vi "ifr2025 Reverse Power Protection  .vi"(8 "error in (no error)":errorcluster {"code" format="%.0x"}, 11 "instrument handle":refnum<visa-resource-name>) -> (0 "error out":errorcluster {"code" format="%.0x"}, 1 "RPP Count":i16, 2 "RPP Tripped":i16, 3 "instrument handle out":refnum<visa-resource-name>)   [LabVIEW 2009]
doc: "Returns information about the reverse power protection circuit."
uses:
  Ifr2025_32.dll
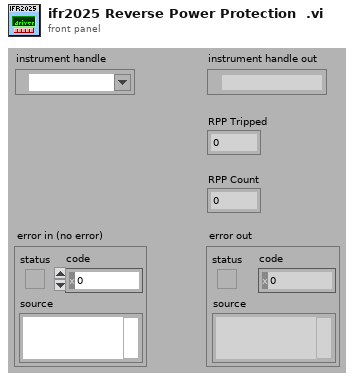
[diagram p1: front panel]
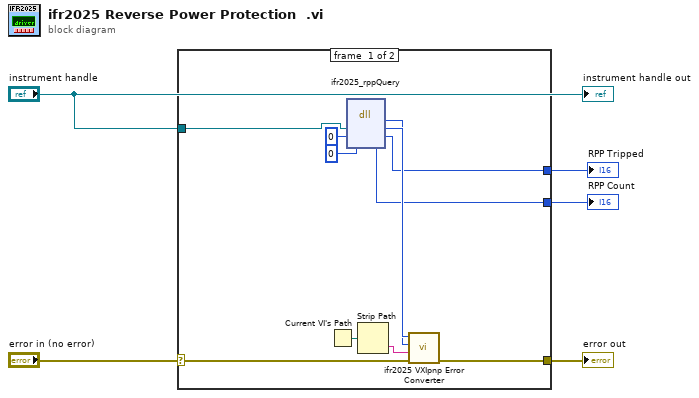
[diagram p0: block diagram]
diagram:
  n1 = case shown="No Error" "error in (no error)" {
    selector: "error in (no error)" -> [w11 w17]
    tunnel: [w10 w17] -> w5
    tunnel: "instrument handle" -> [w15 _]
    tunnel: [w8 _] -> w2
    tunnel: [w6 _] -> w1
    frame #0 {
      n2 = Current VI's Path() -> (path=w16:path)
      n3 = dll-call lib="P:/inst/Marconi 2024 Signal Generator/source/labview/ifr2025/ifr2025/ifr2025_*.*" fn="ifr2025_rppQuery"("vi"=w15, "RPP Tripped"=i16 0, "RPP Count"=i16 0) -> (w13:i32, "vi"=w14:u32, "RPP Tripped"=w8:i16, "RPP Count"=w6:i16)  [unwired: 3 in, 2 out]
      n4 = Strip Path(path=w16) -> (name=w12:string)  [unwired: 1 out]
      n5 = call "ifr2025 VXIpnp Error Converter.vi"("error in (no error)"=w11, "name of VI (\"\")"=w12, "CVI error code (0)"=w13, "instrument handle"=w14) -> ("error out"=w10:errorcluster)  [unwired: 7 out]
    }
    frame #1 {
    }
  }
  "error out" <- w5
  "RPP Tripped" <- w2
  "RPP Count" <- w1
  "instrument handle out" <- "instrument handle"
